vi "Set Double Float.vi"(7 "Name":string="Set Double Float", 10 "Value":dbl, 11 "Abs_Double Float.lvclass":refnum<class "Abs_Double Float.lvclass">) -> (3 "Node":refnum<class "abs_Node.lvclass">)   [LabVIEW 2021, in "BT.lvlib"]
uses:
  BT.lvlib
  Support/abs_Node/abs_Node.lvclass
  <vilib>/TSA/Abstract Data Classes/Abs_Types/Double Float/Abs_Double Float.lvclass
  C:/Program Files (x86)/National Instruments/LabVIEW 2021/vi.lib/TSA/Abstract Data Classes/Abs_Types/Type/Abs_Type.lvclass
  Support/Set Double Float/Set Double Float.lvclass
  C:/Users/Tim/Documents/GitHub/LV_Behaviour_Tree/Source/Support/abs_Type Leaf/abs_Type Leaf.lvclass
  C:/Users/Tim/Documents/GitHub/LV_Behaviour_Tree/Source/Support/abs_Node/abs_Node.lvclass
  Support/abs_Type Leaf/abs_Type Leaf.lvclass/abs_Type Leaf.ctl
  Support/Set Double Float/Set Double Float.lvclass/Set Double Float.ctl
  <vilib>/TSA/Abstract Data Classes/Abs_Types/Type/Abs_Type.lvclass/Abs_Type.ctl
  Support/abs_Type Leaf/Properties/Write Value Class.vi
  Support/Set Double Float/Properties/Write Value.vi
  <vilib>/TSA/Abstract Data Classes/Abs_Types/Type/Properties/Write Name.vi
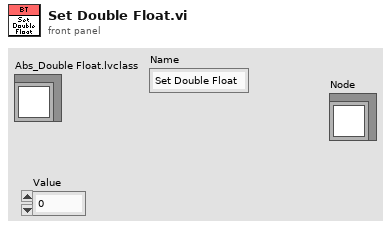
[diagram p1: front panel]
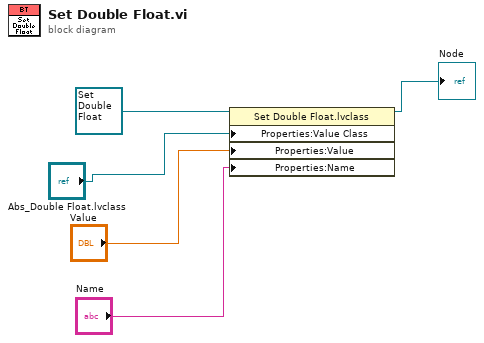
[diagram p0: block diagram]
diagram:
  n1 = property class="Set Double Float.lvclass"(reference=refnum<class "Set Double Float.lvclass"> refnum ("BT.lvlib:Set Double Float.lvclass"), "Properties:Value Class"="Abs_Double Float.lvclass", "Properties:Value"="Value", "Properties:Name"="Name") -> (reference out=→"Node":refnum<class "Set Double Float.lvclass">)  [unwired: 1 in, 1 out]
